vi "TimingTrueAtXHerz.vi"(11 "Graph Update Freuquency (Hz)":u32=5) -> (3 "Boolean":bool)   [LabVIEW 2014]
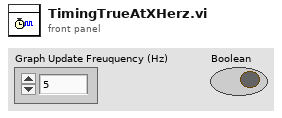
[diagram p1: front panel]
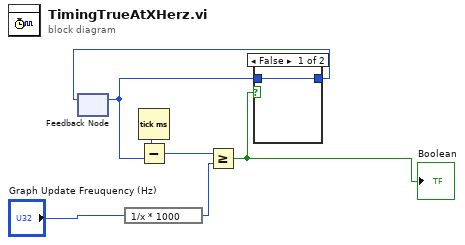
[diagram p0: block diagram]
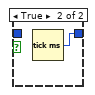
[diagram p2: hidden frame]
diagram:
  n1 = feedback #1() -> (w7:u32)  [unwired: 1 in]
  n2 = expression code="1/x * 1000"("Graph Update Freuquency (Hz)") -> (w3:u32)
  n3 = Tick Count (ms)() -> (millisecond timer value=w4:u32)
  n4 = Subtract(x=w4, y=w7) -> (x-y=w1:u32)
  n5 = Greater Or Equal?(x=w1, y=w3) -> (x >= y?=w5:bool)
  "Boolean" <- w5
  n6 = case shown="False" w5 {
    tunnel: [w8 w9] -> w6
    tunnel: w7 -> [w8 _]
    frame False {
    }
    frame True {
      n7 = Tick Count (ms)() -> (millisecond timer value=w9:u32)
    }
  }
  n8 = feedback-in #1(w6) -> ()
